vi "Switch M83536.vi"() -> ()   [LabVIEW 2014]
panel:
  out "Time to Switch":dbl
  out "End Time":timestamp format="%<%.10X>T"
  out "Stop Ind.":bool
  out "Output On time":timestamp format="%<%.10X>T"
  in  "Output On/Off":bool
  out "Waveform Chart":dynamicdata(graph)
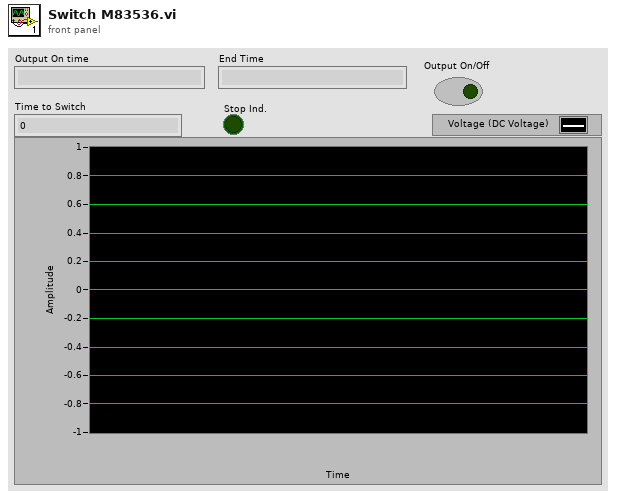
[diagram p1: front panel]
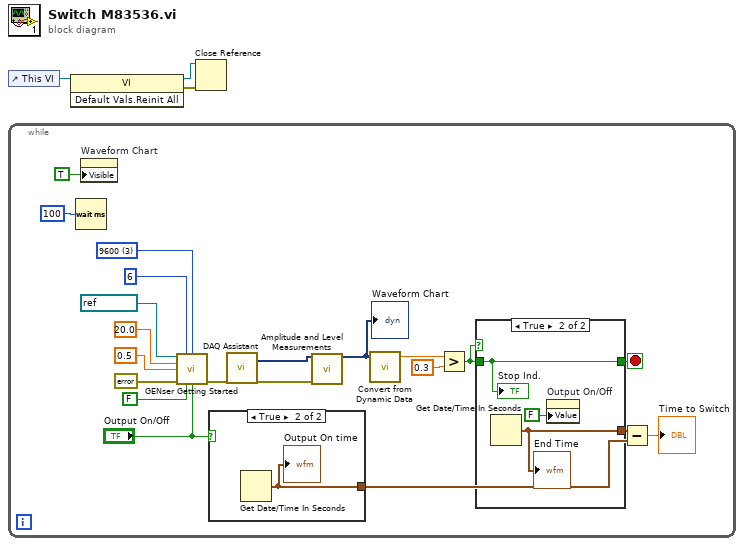
[diagram p0: block diagram]
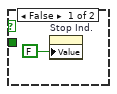
[diagram p2: hidden frame]
diagram:
  n1 = control-ref of="This VI"() -> (w3:refnum<vi>)
  n2 = while {
    stop <- w4 stop-if-true
    w13 = u16 3 items=["1200", "2400", "4800", "9600", "19200"] ("BAUD")
    n3 = Wait (ms)(milliseconds to wait=u32 100) -> ()  [unwired: 1 out]
    n4 = property on="Waveform Chart" class="WFChart (strict)"("Visible"=TRUE) -> ()  [unwired: 2 in, 2 out]
    n5 = call "GENser Getting Started.vi"("VISA"=refnum<visa-resource-name> "COM3", "GEN Addr"=i16 6, "BAUD"=w13, "Voltage Limit"=20.0, "Current Limit"=0.5, "error"=errorcluster {"status"=FALSE, "code"=0, "source"=""}, "Reset (T)"=FALSE, "Output On (T)"="Output On/Off") -> ("error out"=w12:errorcluster)  [unwired: 4 in, 3 out]
    n6 = case shown="True" "Output On/Off" {
      tunnel: [_ w29] -> w7
      frame False {
      }
      frame True {
        n7 = Get Date/Time In Seconds() -> (seconds since 1Jan1904=w29:timestamp)
        "Output On time" <- w29
      }
    }
    n8 = call "DAQ Assistant"("error in"=w12) -> ("data"=w23:dynamicdata, "error out"=w10:errorcluster)  [unwired: 16 in, 1 out]
    n9 = call "Amplitude and Level Measurements"("Signals"=w23, "error in (no error)"=w10) -> ("Mean (DC)"=w22:dynamicdata)  [unwired: 12 in, 1 out]
    "Waveform Chart" <- w22
    n10 = call "Convert from Dynamic Data"("Dynamic Data Type"=w22) -> ("Scalar"=w20:dbl)  [unwired: 3 in]
    n11 = Greater?(x=w20, y=0.3) -> (0:w5:bool)
    n12 = case shown="True" w5 {
      tunnel: [_ w28] -> w6
      tunnel: w5 -> [_ w27]
      tunnel: [_ w27] -> w4
      frame False {
        n13 = property on="Stop Ind." class="Bool (strict)"("Value"=FALSE) -> ()  [unwired: 2 in, 2 out]
      }
      frame True {
        n14 = Get Date/Time In Seconds() -> (seconds since 1Jan1904=w28:timestamp)
        "End Time" <- w28
        n15 = property on="Output On/Off" class="Bool (strict)"("Value"=FALSE) -> ()  [unwired: 2 in, 2 out]
        "Stop Ind." <- w27
      }
    }
    n16 = Subtract(x=w6, y=w7) -> (x-y=→"Time to Switch":dbl)
  }
  n17 = invoke class="VI" method="Default Vals.Reinit All"(reference=w3) -> (reference out=w1:refnum<vi>, error out=w2:errorcluster)  [unwired: 2 in, 1 out]
  n18 = Close Reference(reference=w1, error in (no error)=w2) -> ()  [unwired: 1 out]
